vi "Override Error.vi"(10 "Error":errorcluster, 11 "Base Actor in":refnum<class "Base Actor.lvclass">) -> (3 "Base Actor out":refnum<class "Base Actor.lvclass">)   [LabVIEW 2021, in "jettl.lvlib" / "Actor.lvlib" / "Base Actor.lvclass"]
uses:
  Base Actor.lvclass
  Base Actor.lvclass/Base Actor.ctl
  State.ctl
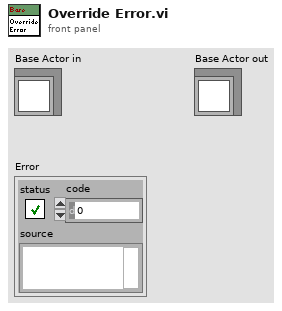
[diagram p1: front panel]
types:
  T1 = typedef "jettl.lvlib/Actor.lvlib/Base Actor.lvclass/State.ctl" = enum16{"Nominal", "Teardown", "Error"}
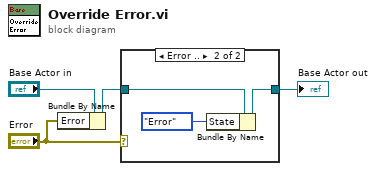
[diagram p0: block diagram]
diagram:
  n1 = Bundle By Name(cluster="Base Actor in", "Error"="Error") -> (w3:refnum<class "Base Actor.lvclass">)
  n2 = case shown="Error .." "Error" {
    tunnel: [w5 w7] -> w2
    tunnel: w3 -> [w5 w8]
    frame No Error {
    }
    frame Error {
      n3 = Bundle By Name(cluster=w8, "State"=State."Error") -> (w7:refnum<class "Base Actor.lvclass">)
    }
  }
  "Base Actor out" <- w2
